vi "测试.vi"() -> ()   [LabVIEW 2011]
uses:
  <vilib>/Utility/miscctls.llb/LVPointDoubleTypeDef.ctl
panel:
  in  "端点C":T1={"X"=200.0, "Y"=50.0} caption="点"
  out "Picture":picture caption="图片"
  in  "端点B":T1={"X"=150.0, "Y"=150.0} caption="点"
  in  "端点A":T1={"X"=50.0, "Y"=50.0} caption="点"
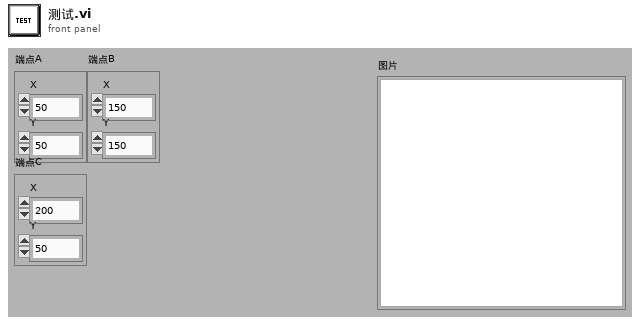
[diagram p1: front panel]
types:
  T1 = typedef "LVPointDoubleTypeDef.ctl" = cluster{"X":dbl, "Y":dbl}
  T2 = cluster{"Width":u16, "Style":enum32{"Solid", "Dash", "Dot", "DashDot", "DashDotDot"}}
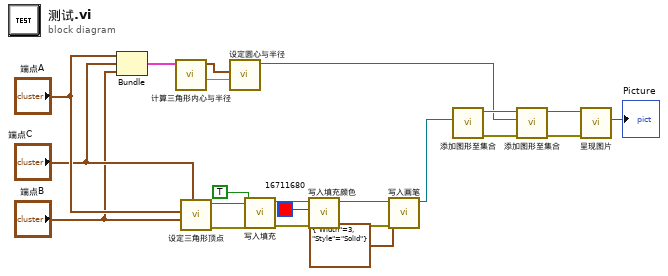
[diagram p0: block diagram]
diagram:
  n1 = Bundle("端点A"="端点A", "端点C"="端点C", "端点B"="端点B") -> (w11:cluster{"端点A":T1, "端点C":T1, "端点B":T1})  [unwired: 1 in]
  n2 = call "计算三角形内心与半径.vi"("三角形"=w11) -> ("半径"=w16:dbl, "内心"=w15:T1)  [unwired: 9 in]
  n3 = call "设定三角形顶点.vi"("端点C"="端点C", "端点B"="端点B", "端点A"="端点A") -> ("error out"=w9:errorcluster, "三角形 输出"=w10:refnum<class "三角形.lvclass">)  [unwired: 7 in]
  n4 = call "设定圆心与半径.vi"("半径"=w16, "圆心"=w15) -> ("圆形 输出"=w19:refnum<class "圆形.lvclass">)  [unwired: 8 in, 1 out]
  n5 = call "写入填充.vi"("error in (no error)"=w9, "填充"=TRUE, "图形输入"=w10) -> ("error out"=w5:errorcluster, "图形输出"=w7:refnum<class "三角形.lvclass">)  [unwired: 7 in]
  n6 = call "写入填充颜色.vi"("error in (no error)"=w5, "填充颜色"=u32 16711680, "图形输入"=w7) -> ("error out"=w4:errorcluster, "图形输出"=w6:refnum<class "三角形.lvclass">)  [unwired: 7 in]
  n7 = call "写入画笔.vi"("error in (no error)"=w4, "画笔"=T2 {"Width"=3, "Style"=enum."Solid"}, "图形输入"=w6) -> ("图形输出"=w1:refnum<class "三角形.lvclass">)  [unwired: 7 in, 1 out]
  n8 = call "添加图形至集合.vi"("图形.lvclass"=w1) -> ("error out"=w21:errorcluster, "集合 输出"=w20:refnum<class "集合.lvclass">)  [unwired: 9 in]
  n9 = call "添加图形至集合.vi"("error in (no error)"=w21, "图形.lvclass"=w19, "集合 输入"=w20) -> ("error out"=w17:errorcluster, "集合 输出"=w18:refnum<class "集合.lvclass">)  [unwired: 7 in]
  n10 = call-dynamic "呈现图片.vi"("error in (no error)"=w17, "集合 输入"=w18) -> ("Picture"=→"Picture":picture)  [unwired: 7 in, 2 out]
